vi "Update Table.vi"(8 "error in (no error)":errorcluster, 10 "Table":refnum<class "Basic Table.lvclass">, 11 "Panel Form Controller in":refnum<class "Panel Form Controller.lvclass">) -> (0 "error out":errorcluster, 3 "Panel Form Controller out":refnum<class "Panel Form Controller.lvclass">)   [LabVIEW 2020, in "Panel Form Controller.lvlib" / "Panel Form Controller.lvclass"]
uses:
  Panel Form Controller.lvclass
  Database OOP/Table Libraries/Basic Table/Basic Table Class/Basic Table.lvclass
  Panel Form Controller.lvclass/Panel Form Controller.ctl
  Database OOP/Table Libraries/Basic Form/Basic Form.lvclass
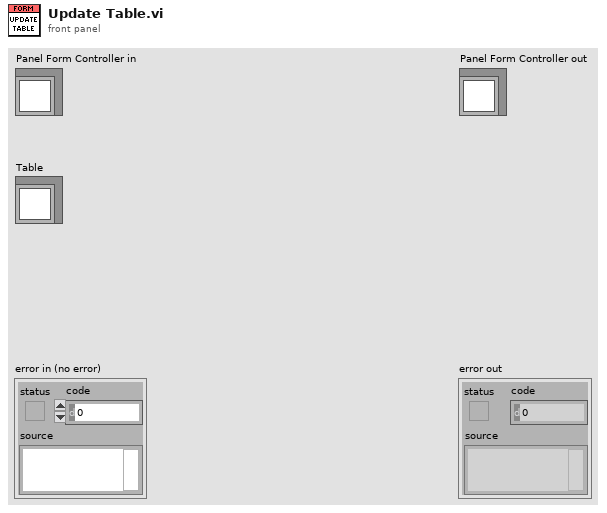
[diagram p1: front panel]
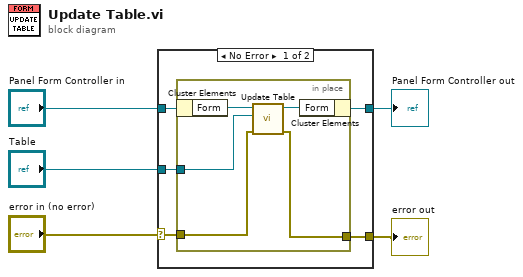
[diagram p0: block diagram]
diagram:
  n1 = case shown="No Error" "error in (no error)" {
    selector: "error in (no error)" -> [w8 w17]
    tunnel: [w6 w17] -> w4
    tunnel: [w9 w16] -> w2
    tunnel: "Panel Form Controller in" -> [w10 w16]
    tunnel: "Table" -> [w7 _]
    frame No Error {
      n2 = in-place {
        in-place-border: w8 -> [w12]
        in-place-border: w7 -> [w14]
        in-place-border: [w11] -> w6
        n3 = in-place-cluster #1(w10) -> ("Form"=w15:refnum<class "Basic Form.lvclass">)
        n4 = call-dynamic "Update Table.vi"("error in (no error)"=w12, "New Values Table"=w14, "Basic Table in"=w15) -> ("error out"=w11:errorcluster, "Basic Table out"=w13:refnum<class "Basic Form.lvclass">)  [unwired: 7 in]
        n5 = in-place-cluster #1("Form"=w13) -> (w9:refnum<class "Panel Form Controller.lvclass">)
      }
    }
    frame Error {
    }
  }
  "error out" <- w4
  "Panel Form Controller out" <- w2
